vi "Save User.vi"(8 "error in (no error)":errorcluster, 10 "User In":refnum<class "SOL User.lvclass">, 11 "User DB in":refnum<class "User DB.lvclass">) -> (0 "error out":errorcluster, 2 "User":refnum<class "SOL User.lvclass">, 3 "User DB out":refnum<class "User DB.lvclass">)   [LabVIEW 2020, in "Summer of LabVIEW.lvlib" / "User DB.lvclass"]
uses:
  User DB.lvclass
  SOL User/SOL User.lvclass
  User DB.lvclass/User DB.ctl
  <vilib>/drjdpowell/SQLite Library/SQL Statement/SQL Statement.lvclass/SQL Statement.ctl
  <vilib>/drjdpowell/SQLite Library/SQL Connection/Connection.lvclass/Connection.ctl
  <vilib>/drjdpowell/SQLite Library/SQL Statement/Bind Integer.vi
  <vilib>/drjdpowell/SQLite Library/SQL Statement/Bind Text.vi
  <vilib>/drjdpowell/SQLite Library/SQL Statement/Step.vi
  <vilib>/drjdpowell/SQLite Library/SQL Statement/Error Message.vi
  SQLite/SQLite.lvclass
  <vilib>/drjdpowell/SQLite Library/SQL Connection/Connection.lvclass
  <vilib>/drjdpowell/SQLite Library/SQL Statement/SQL Statement.lvclass
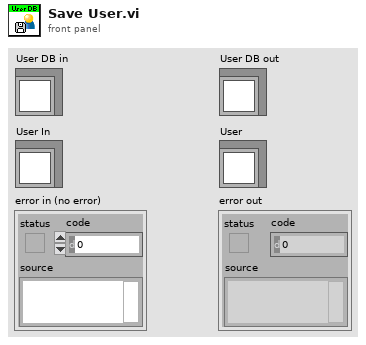
[diagram p1: front panel]
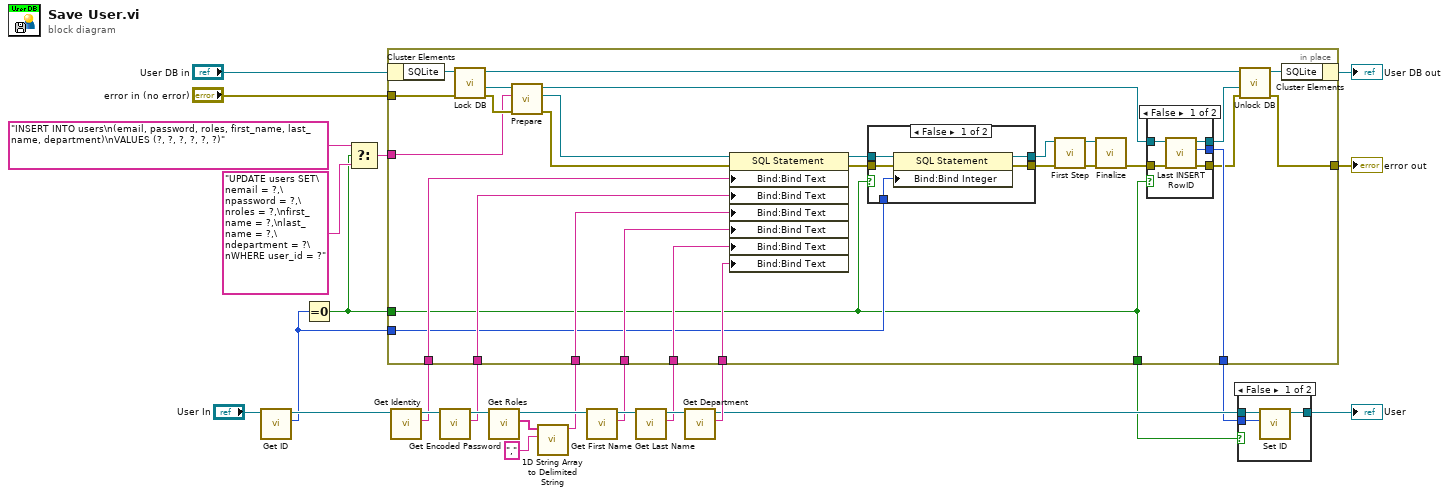
[diagram p0: block diagram]
diagram:
  n1 = call "Get ID.vi"("SOL User in"="User In") -> ("ID"=w8:i64, "SOL User out"=w19:refnum<class "SOL User.lvclass">)  [unwired: 8 in, 1 out]
  n2 = Equal To 0?(x=w8) -> (x = 0?=w7:bool)
  n3 = Select(t="INSERT INTO users\n(email, password, roles, first_name, last_name, department)\nVALUES (?, ?, ?, ?, ?, ?)" ("SQL"), s=w7, f="UPDATE users SET\nemail = ?,\npassword = ?,\nroles = ?,\nfirst_name = ?,\nlast_name = ?,\ndepartment = ?\nWHERE user_id = ?" ("SQL")) -> (s? t:f=w15:string)
  n4 = call-dynamic "Get Identity.vi"("SOL User in"=w19) -> ("Identity"=w14:string, "SOL User out"=w28:refnum<class "SOL User.lvclass">)  [unwired: 8 in, 1 out]
  n5 = call-dynamic "Get Encoded Password.vi"("SOL User in"=w28) -> ("Encoded Password"=w13:string, "SOL User out"=w27:refnum<class "SOL User.lvclass">)  [unwired: 8 in, 1 out]
  n6 = call-dynamic "Get Roles.vi"("SOL User in"=w27) -> ("Roles"=w26:string[], "SOL User out"=w24:refnum<class "SOL User.lvclass">)  [unwired: 8 in, 1 out]
  n7 = call <vilib>:"1D String Array to Delimited String.vi"("delimiter"=",", "string array"=w26) -> ("delimited string"=w12:string)  [unwired: 9 in]
  n8 = call "Get First Name.vi"("SOL User in"=w24) -> ("First Name"=w11:string, "SOL User out"=w23:refnum<class "SOL User.lvclass">)  [unwired: 8 in, 1 out]
  n9 = call "Get Last Name.vi"("SOL User in"=w23) -> ("Last Name"=w10:string, "SOL User out"=w22:refnum<class "SOL User.lvclass">)  [unwired: 8 in, 1 out]
  n10 = call "Get Department.vi"("SOL User in"=w22) -> ("Department"=w9:string, "SOL User out"=w6:refnum<class "SOL User.lvclass">)  [unwired: 8 in, 1 out]
  n11 = in-place {
    in-place-border: "error in (no error)" -> [w55]
    in-place-border: w15 -> [w53]
    in-place-border: w14 -> [w50]
    in-place-border: w13 -> [w49]
    in-place-border: w12 -> [w48]
    in-place-border: w11 -> [w47]
    in-place-border: w10 -> [w46]
    in-place-border: w9 -> [w45]
    in-place-border: w8 -> [w42]
    in-place-border: w7 -> [w31]
    in-place-border: [w32] -> w5
    in-place-border: [w31] -> w4
    in-place-border: [w29] -> w1
    n12 = in-place-cluster #1("User DB in") -> ("SQLite"=w57:refnum<class "SQLite.lvclass">)
    n13 = call "Lock DB.vi"("error in (no error)"=w55, "SQLite in"=w57) -> ("error out"=w54:errorcluster, "SQLite DB"=w56:refnum<class "Connection.lvclass">, "SQLite out"=w35:refnum<class "SQLite.lvclass">)  [unwired: 6 in, 1 out]
    n14 = call <vilib>:"Prepare.vi"("error in (no error)"=w54, "SQL"=w53, "SQLite Connection in"=w56) -> ("error out"=w52:errorcluster, "SQL Statement"=w51:refnum<class "SQL Statement.lvclass">, "SQLite Connection"=w36:refnum<class "Connection.lvclass">)  [unwired: 4 in, 2 out]
    n15 = property class="SQL Statement"(reference=w51, error in=w52, "Bind:Bind Text"=w50, "Bind:Bind Text"=w49, "Bind:Bind Text"=w48, "Bind:Bind Text"=w47, "Bind:Bind Text"=w46, "Bind:Bind Text"=w45) -> (reference out=w44:refnum<class "SQL Statement.lvclass">, error out=w43:errorcluster)
    n16 = case shown="False" w31 {
      tunnel: w44 -> [w69 w71]
      tunnel: w43 -> [w68 w70]
      tunnel: w42 -> [w67 _]
      tunnel: [w66 w71] -> w40
      tunnel: [w65 w70] -> w41
      frame False {
        n17 = property class="SQL Statement"(reference=w69, error in=w68, "Bind:Bind Integer"=w67) -> (reference out=w66:refnum<class "SQL Statement.lvclass">, error out=w65:errorcluster)
      }
      frame True {
      }
    }
    n18 = call <vilib>:"First Step.vi"("error in (no error)"=w41, "SQL Statement in"=w40) -> ("error out"=w39:errorcluster, "SQL Statement"=w38:refnum<class "SQL Statement.lvclass">)  [unwired: 7 in, 1 out]
    n19 = call <vilib>:"Finalize.vi"("error in (no error)"=w39, "SQL Statement in"=w38) -> ("error out"=w37:errorcluster)  [unwired: 9 in]
    n20 = case shown="False" w31 {
      tunnel: w37 -> [w62 w63]
      tunnel: w36 -> [w61 w64]
      tunnel: [w60 w64] -> w34
      tunnel: [w59 _] -> w32
      tunnel: [w58 w63] -> w30
      frame False {
        n21 = call <vilib>:"Last INSERT RowID.vi"("error in (no error)"=w62, "SQLite Connection in"=w61) -> ("error out"=w58:errorcluster, "Last INSERT RowID"=w59:i64, "SQLite Connection"=w60:refnum<class "Connection.lvclass">)  [unwired: 7 in]
      }
      frame True {
      }
    }
    n22 = call "Unlock DB.vi"("error in (no error)"=w30, "SQLite DB"=w34, "SQLite in"=w35) -> ("error out"=w29:errorcluster, "SQLite out"=w33:refnum<class "SQLite.lvclass">)  [unwired: 7 in]
    n23 = in-place-cluster #1("SQLite"=w33) -> (→"User DB out":refnum<class "User DB.lvclass">)
  }
  "error out" <- w1
  n24 = case shown="False" w4 {
    tunnel: w6 -> [w74 w75]
    tunnel: w5 -> [w73 _]
    tunnel: [w72 w75] -> w3
    frame False {
      n25 = call "Set ID.vi"("ID"=w73, "SOL User in"=w74) -> ("SOL User out"=w72:refnum<class "SOL User.lvclass">)  [unwired: 8 in, 1 out]
    }
    frame True {
    }
  }
  "User" <- w3
